vi "Get LTS Stage Position.vi"(8 "error in (no error)":errorcluster, 10 "Cluster in":T1, 11 "LTS Reference In":refnum<k24>) -> (0 "error out":errorcluster, 1 "GetMoveAbsolutePosition":dbl, 2 "Cluster out":T1, 3 "LTS Reference Out":refnum<k24>)   [LabVIEW 2014]
uses:
  Ctrls/Translation Stage Cluster.ctl
  C:/Projects/Serial Sectioning OCT - TortoiseGIT/SerialSectOCT/Software/Test Code/Thorlabs.MotionControl.Controls.dll
  Thorlabs.MotionControl.Controls.dll
  C:/Projects/Serial Sectioning OCT - TortoiseGIT/SerialSectOCT/Software/Thorlabs.MotionControl.IntegratedStepperMotorsCLI.dll
  Thorlabs.MotionControl.IntegratedStepperMotorsCLI.dll
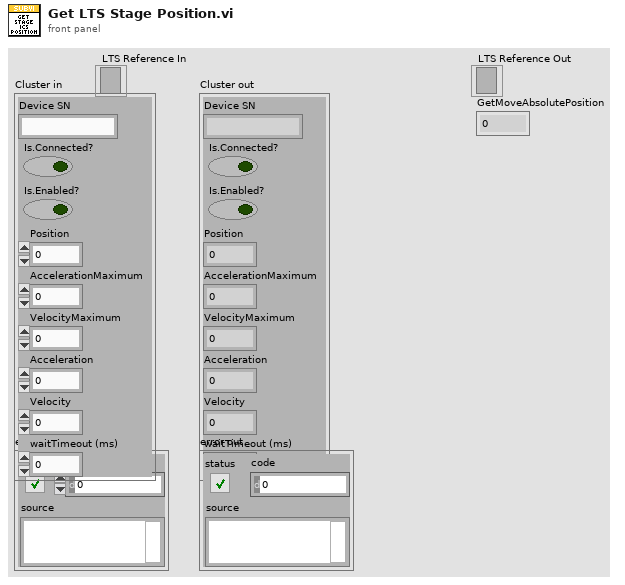
[diagram p1: front panel]
types:
  T1 = typedef "Translation Stage Cluster.ctl" = cluster{"Device SN":string, "Is.Connected?":bool, "Is.Enabled?":bool, "Position":dbl, "AccelerationMaximum":dbl, "VelocityMaximum":dbl, "Acceleration":dbl, "Velocity":dbl, "waitTimeout (ms)":i32}
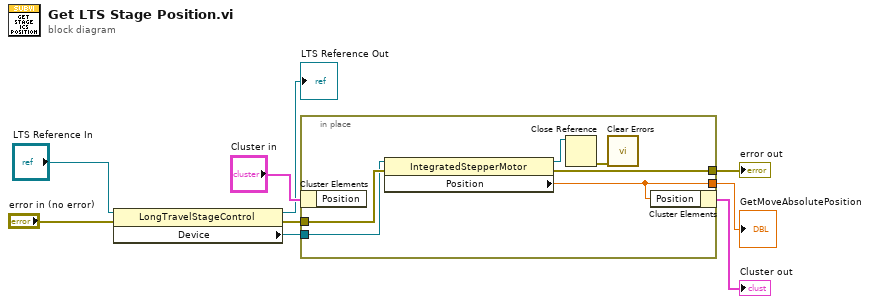
[diagram p0: block diagram]
diagram:
  n1 = property class="LongTravelStageControl"(reference="LTS Reference In", error in="error in (no error)") -> (reference out=→"LTS Reference Out":refnum<k24>, error out=w2:errorcluster, "Device"=w1:refnum<k24>)
  n2 = in-place {
    in-place-border: [w15] -> w7
    in-place-border: [w12] -> w6
    in-place-border: w2 -> [w11]
    in-place-border: w1 -> [w10]
    n3 = in-place-cluster #1("Cluster in") -> ()  [unwired: 1 out]
    n4 = property class="IntegratedStepperMotor"(reference=w10, error in=w11) -> (reference out=w13:refnum<k24>, error out=w15:errorcluster, "Position"=w12:dbl)
    n5 = Close Reference(reference=w13) -> (error out=w14:errorcluster)  [unwired: 1 in]
    n6 = call <vilib>:"Clear Errors.vi"("error in (no error)"=w14) -> ()  [unwired: 5 in, 2 out]
    n7 = in-place-cluster #1("Position"=w12) -> (→"Cluster out":T1)
  }
  "error out" <- w7
  "GetMoveAbsolutePosition" <- w6
